vi "OOP_UP.vi"(8 "error in (no error)":errorcluster, 10 "Sett data":T2={"Filter"=4, "Gain"=4.0, "Bit rate"=4.0, "ISO/IEC w "=enum."14443 Type A", "BI"={"R"=0.0, "C"=0.0, "L"=0.0}, "BM"={"R"=0.0, "C"=0.0, "L"=0.0}, "M"={"Метка"=4, "Считыветель"=4}, "Type noise"=enum."Гауссовский шум", "Link"=enum."UPLINK", "Noise attenuator"=0.0, "Signal gain"=1.0, "Distance"=0.0} {"Distance" scale=0.0..10.0; "Signal gain" min=1.0 max=100.0 step=1.0 scale=1.0..30.0; "Noise attenuator" scale=0.01..1.01; "M"."Считыветель" min=4 max=128 step=4; "M"."Метка" min=4 max=128 step=4; "Bit rate" min=4.0 max=128.0 step=4.0; "Gain" min=4.0 max=128.0 step=4.0; "Filter" min=4 max=128 step=4}, 11 "RFID system in":refnum<class "RFID system.lvclass">) -> (0 "error out":errorcluster, 2 "Error on  byte":dbl, 3 "Visual":T1)   [LabVIEW 2019]
uses:
  Class/RFID system.lvclass
  TypeDef/Sett data.ctl
  TypeDef/ISO.ctl
  TypeDef/Noise.ctl
  TypeDef/Link.ctl
  UI/Visual/data.ctl
  TypeDef/Store.ctl
  UI/Visual/Visual.xctl
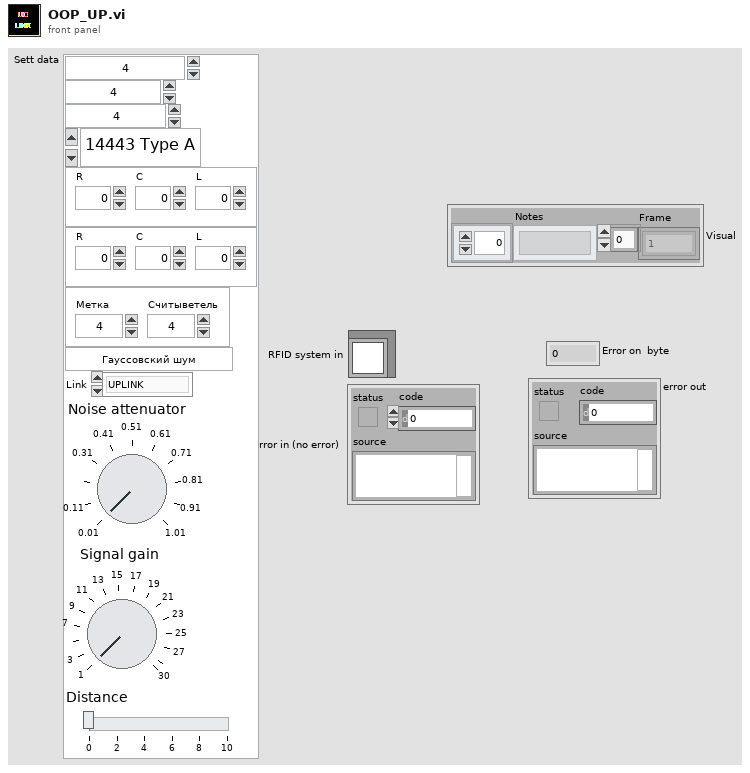
[diagram p1: front panel]
types:
  T1 = typedef "Visual.xctl/data.ctl" = cluster{"Notes":string[], "Frame":u8[]}
  T2 = typedef "Sett data.ctl" = cluster{"Filter":i32, "Gain":dbl, "Bit rate":dbl, "ISO/IEC w ":T3, "BI":cluster{"R":dbl, "C":dbl, "L":dbl}, "BM":cluster{"R":dbl, "C":dbl, "L":dbl}, "M":cluster{"Метка":i64, "Считыветель":i64}, "Type noise":T4, "Link":T5, "Noise attenuator":dbl, "Signal gain":dbl, "Distance":dbl}
  T3 = typedef "ISO.ctl" = enum16{"14443 Type A", "14443 Type B", "Felica", "15693"}
  T4 = typedef "Noise.ctl" = enum16{"Гауссовский шум", "Белый шум"}
  T5 = typedef "Link.ctl" = enum16{"UPLINK", "DOWNLINK"}
  T6 = typedef "Store.ctl" = enum16{"envelope", "noise", "demSubCar", "CH_frame", "Decode", "demodulate", "in", "out", "sum", "subCarrier", "frame", "command", "encode", "modulate", "encode_UP", "modulate_up", "demod_up", "envelop_up", "sum_up", "out_up", "in_up"}
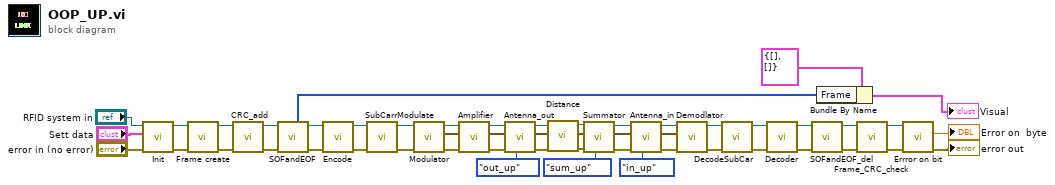
[diagram p0: block diagram]
diagram:
  n1 = call "Init.vi"("error in (no error)"="error in (no error)", "Sett data"="Sett data", "RFID system in"="RFID system in") -> ("error out"=w51:errorcluster, "RFID system out"=w50:refnum<class "RFID system.lvclass">)  [unwired: 7 in]
  n2 = call-dynamic "Frame create.vi"("error in (no error)"=w51, "RFID system in"=w50) -> ("error out"=w49:errorcluster, "RFID system out"=w48:refnum<class "RFID system.lvclass">)  [unwired: 8 in]
  n3 = call-dynamic "CRC_add.vi"("error in (no error)"=w49, "RFID system in"=w48) -> ("error out"=w46:errorcluster, "RFID system out"=w47:refnum<class "RFID system.lvclass">)  [unwired: 8 in]
  n4 = call-dynamic "SOFandEOF.vi"("error in (no error)"=w46, "RFID system in"=w47) -> ("error out"=w39:errorcluster, "RFID system out"=w40:refnum<class "RFID system.lvclass">, "frame"=w1:u8[])  [unwired: 7 in]
  n5 = call-dynamic "Encode.vi"("error in (no error)"=w39, "RFID system in"=w40) -> ("error out"=w37:errorcluster, "RFID system out"=w38:refnum<class "RFID system.lvclass">)  [unwired: 8 in]
  n6 = call-dynamic "SubCarrModulate.vi"("error in (no error)"=w37, "RFID system in"=w38) -> ("error out"=w35:errorcluster, "RFID system out"=w36:refnum<class "RFID system.lvclass">)  [unwired: 8 in]
  n7 = call-dynamic "Modulator.vi"("error in (no error)"=w35, "RFID system in"=w36) -> ("error out"=w32:errorcluster, "Waveform out"=w34:waveform(dbl), "RFID system out"=w33:refnum<class "RFID system.lvclass">)  [unwired: 7 in]
  n8 = call "Amplifier.vi"("error in (no error)"=w32, "Waveform in"=w34, "RFID system in"=w33) -> ("error out"=w30:errorcluster, "Waveform out"=w29:waveform(dbl), "RFID system out"=w31:refnum<class "RFID system.lvclass">)  [unwired: 6 in]
  n9 = call "Antenna_out.vi"("Store"=Store."out_up", "error in (no error)"=w30, "Waveform in"=w29, "RFID system in"=w31) -> ("error out"=w10:errorcluster, "Waveform out"=w11:waveform(dbl), "RFID system out"=w12:refnum<class "RFID system.lvclass">)  [unwired: 5 in]
  n10 = call "Distance.vi"("error in (no error)"=w10, "Waveform in"=w11, "RFID system in"=w12) -> ("error out"=w9:errorcluster, "Waveform out"=w8:waveform(dbl), "RFID system out"=w7:refnum<class "RFID system.lvclass">)  [unwired: 6 in]
  n11 = call "Summator.vi"("Store"=Store."sum_up", "error in (no error)"=w9, "Waveform in"=w8, "RFID system in"=w7) -> ("error out"=w4:errorcluster, "Waveform out"=w5:waveform(dbl), "RFID system out"=w6:refnum<class "RFID system.lvclass">)  [unwired: 5 in]
  n12 = call "Antenna_in.vi"("Store"=Store."in_up", "error in (no error)"=w4, "Waveform in"=w5, "RFID system in"=w6) -> ("error out"=w27:errorcluster, "Waveform out"=w26:waveform(dbl), "RFID system out"=w28:refnum<class "RFID system.lvclass">)  [unwired: 5 in]
  n13 = call-dynamic "Demodlator.vi"("error in (no error)"=w27, "Waveform in"=w26, "RFID system in"=w28) -> ("error out"=w24:errorcluster, "RFID system out"=w25:refnum<class "RFID system.lvclass">)  [unwired: 6 in, 1 out]
  n14 = call-dynamic "DecodeSubCar.vi"("error in (no error)"=w24, "RFID system in"=w25) -> ("error out"=w22:errorcluster, "RFID system out"=w23:refnum<class "RFID system.lvclass">)  [unwired: 8 in]
  n15 = call-dynamic "Decoder.vi"("error in (no error)"=w22, "RFID system in"=w23) -> ("error out"=w20:errorcluster, "RFID system out"=w21:refnum<class "RFID system.lvclass">)  [unwired: 8 in]
  n16 = call-dynamic "SOFandEOF_del.vi"("error in (no error)"=w20, "RFID system in"=w21) -> ("error out"=w18:errorcluster, "RFID system out"=w19:refnum<class "RFID system.lvclass">)  [unwired: 8 in]
  n17 = Bundle By Name(cluster=T1 {"Notes"=[], "Frame"=[]} ("Store"), "Frame"=w1) -> (→"Visual":T1)
  n18 = call-dynamic "Frame_CRC_check.vi"("error in (no error)"=w18, "RFID system in"=w19) -> ("error out"=w17:errorcluster, "RFID system out"=w16:refnum<class "RFID system.lvclass">)  [unwired: 8 in]
  n19 = call-dynamic "Errror on bit.vi"("error in (no error)"=w17, "RFID system in"=w16) -> ("error out"=→"error out":errorcluster, "Error on  byte"=→"Error on  byte":dbl)  [unwired: 7 in, 1 out]
